vi "周期设置_多参数.vi"() -> ()   [LabVIEW 2016, in "斯坦道多参数.lvlib"]
uses:
  <vilib>/Utility/miscctls.llb/LVPointTypeDef.ctl
  <vilib>/Utility/config.llb/NI_LVConfig.lvlib
panel:
  in  "运行周期":T1
  # "运行模式："
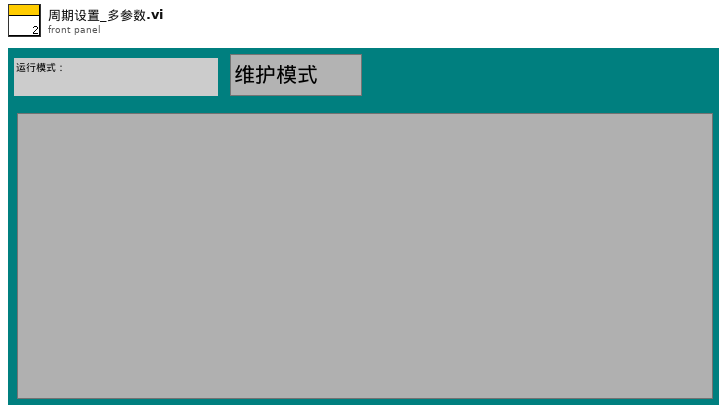
[diagram p1: front panel]
types:
  T1 = cluster{"运行模式":enum16{"维护模式", "常规模式", "应急模式", "质控模式"}, "24H周期设置":bool[]}
  T2 = typedef "斯坦道多参数.lvlib/水样测试启动自定义输入参数.ctl" = cluster{"测量模式":enum16{"待机", "水样测试", "标样核查", "零点核查", "跨度核查", "空白测试", "平行样测试", "加标回收", "空白校准", "标样校准", "初始化（清洗）"}, "数据类型":string, "手动启动标记":bool}
  T3 = typedef "LVPointTypeDef.ctl" = cluster{"Horizontal":i16, "Vertical":i16}
  T4 = typedef "NI_LVConfig.lvlib/Config Data RefNum.ctl" = refnum<k1>
  T5 = typedef "LVDateTimeRec.ctl" = cluster{"秒数的小数部分":dbl, "秒":i32, "分":i32, "时":i32, "日":i32, "月":i32, "年":i32, "天数（周）":i32, "天数（年）":i32, "DST":i32}
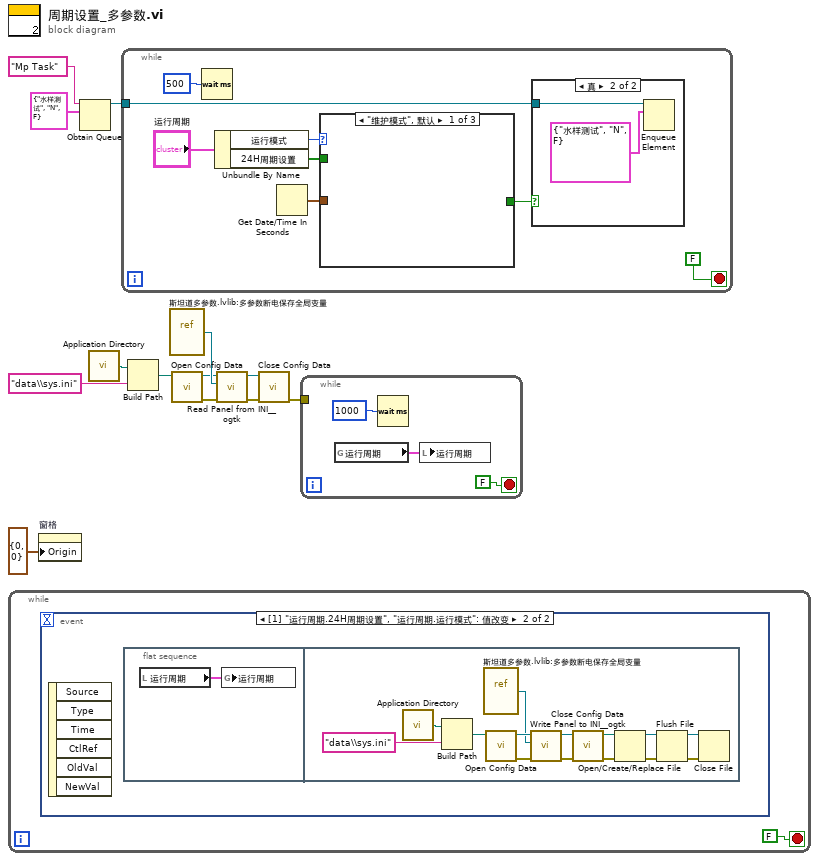
[diagram p0: block diagram]
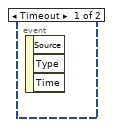
[diagram p2: hidden frame]
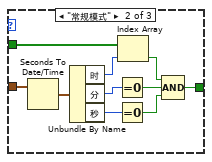
[diagram p4: hidden frame]
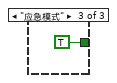
[diagram p5: hidden frame]
diagram:
  n1 = while {
    stop <- FALSE stop-if-true
    n2 = event shown="[1] \"运行周期.24H周期设置\", \"运行周期.运行模式\": 值改变" {
      selector: _ -> [_ _]
      dyn-events: _ -> [_ _]
      timeout: _ -> [_ _]
      event Timeout {
        n3 = event-data() -> ()  [unwired: 1 in, 3 out]
      }
      event "运行周期.24H周期设置", "运行周期.运行模式": Value Change {
        n4 = event-data() -> ()  [unwired: 1 in, 6 out]
        n5 = flat-sequence {
          frame #0 {
            n6 = local read "运行周期"() -> (w15:T1)
            n7 = global write "多参数断电保存全局变量.vi" "运行周期"(w15) -> ()
          }
          frame #1 {
            n8 = call <vilib>:"Application Directory.vi"() -> ("Application Directory"=w29:path)
            n9 = Build Path(base path=w29, name or relative path="data\\sys.ini" ("名称或相对路径")) -> (appended path=w27:path)
            n10 = vi-ref "斯坦道多参数.lvlib:多参数断电保存全局变量.vi"() -> (w25:refnum<vi>)
            n11 = call <vilib>:"Open Config Data.vi"("configuration file path"=w27) -> ("error out"=w23:errorcluster, "refnum"=w26:T4)  [unwired: 8 in, 1 out]
            n12 = call <userlib>:"Write Panel to INI__ogtk.vi"("error in (no error)"=w23, "VI ref"=w25, "refnum"=w26) -> ("error out"=w22:errorcluster, "refnum out"=w24:T4)  [unwired: 7 in]
            n13 = call <vilib>:"Close Config Data.vi"("error in (no error)"=w22, "refnum"=w24) -> ("error out"=w17:errorcluster, "file path"=w16:path)  [unwired: 8 in]
            n14 = Open/Create/Replace File(file path (use dialog)=w16, error in=w17) -> (refnum out=w20:refnum<file>, error out=w21:errorcluster)  [unwired: 4 in, 1 out]
            n15 = Flush File(refnum=w20, error in=w21) -> (refnum out=w19:refnum<file>, error out=w18:errorcluster)
            n16 = Close File(refnum=w19, error in=w18) -> ()  [unwired: 2 out]
          }
        }
      }
    }
  }
  n17 = property on="窗格" class="Pane"("Origin"=T3 {"Horizontal"=0, "Vertical"=0} ("原点")) -> ()  [unwired: 2 in, 2 out]
  n18 = Obtain Queue(name (unnamed)="Mp Task" ("名称（未命名）"), element data type=T2 {"测量模式"=enum."水样测试", "数据类型"="N", "手动启动标记"=FALSE} ("启动参数")) -> (queue out=w1:refnum<queue>)  [unwired: 3 in, 2 out]
  n19 = call <vilib>:"Application Directory.vi"() -> ("Application Directory"=w6:path)
  n20 = while {
    tunnel: w1 -> [w30]
    stop <- FALSE stop-if-true
    n21 = Wait (ms)(milliseconds to wait=u32 500 ("等待时间（毫秒）")) -> ()  [unwired: 1 out]
    n22 = Unbundle By Name("运行周期") -> ("运行模式"=w31:enum16{"维护模式", "常规模式", "应急模式", "质控模式"}, "24H周期设置"=w33:bool[])
    n23 = Get Date/Time In Seconds() -> (seconds since 1Jan1904=w37:timestamp)
    n24 = case shown="\"维护模式\", 默认" w31 {
      tunnel: w37 -> [_ w49 _]
      tunnel: w33 -> [_ w46 _]
      tunnel: [_ w40 TRUE] -> w32
      frame "维护模式", Default {
      }
      frame "常规模式" {
        n25 = Seconds To Date/Time(time stamp (now)=w49) -> (date time rec=w48:T5)  [unwired: 1 in]
        n26 = Unbundle By Name(w48) -> ("时"=w47:i32, "分"=w45:i32, "秒"=w44:i32)
        n27 = Equal To 0?(x=w45) -> (x = 0?=w42:bool)
        n28 = Equal To 0?(x=w44) -> (x = 0?=w41:bool)
        n29 = Index Array(array=w46, index=w47) -> (element=w43:bool)
        n30 = Compound Arithmetic op=AND ("复合运算")(w43, w42, w41) -> (w40:bool)
      }
      frame "应急模式" {
      }
    }
    n31 = case shown="真" w32 {
      tunnel: w30 -> [_ w39]
      frame False {
      }
      frame True {
        n32 = Enqueue Element(queue=w39, element=T2 {"测量模式"=enum."水样测试", "数据类型"="N", "手动启动标记"=FALSE} ("启动参数")) -> ()  [unwired: 2 in, 3 out]
      }
    }
  }
  n33 = Build Path(base path=w6, name or relative path="data\\sys.ini" ("名称或相对路径")) -> (appended path=w8:path)
  n34 = vi-ref "斯坦道多参数.lvlib:多参数断电保存全局变量.vi"() -> (w10:refnum<vi>)
  n35 = call <vilib>:"Open Config Data.vi"("configuration file path"=w8) -> ("error out"=w12:errorcluster, "refnum"=w9:T4)  [unwired: 8 in, 1 out]
  n36 = call <userlib>:"Read Panel from INI__ogtk.vi"("error in (no error)"=w12, "VI ref"=w10, "refnum"=w9) -> ("error out"=w13:errorcluster, "refnum out"=w11:T4)  [unwired: 7 in]
  n37 = call <vilib>:"Close Config Data.vi"("error in (no error)"=w13, "refnum"=w11) -> ("error out"=w5:errorcluster)  [unwired: 8 in, 1 out]
  n38 = while {
    tunnel: w5 -> [_]
    stop <- FALSE stop-if-true
    n39 = global read "多参数断电保存全局变量.vi" "运行周期"() -> (w51:T1)
    n40 = Wait (ms)(milliseconds to wait=u32 1000 ("等待时间（毫秒）")) -> ()  [unwired: 1 out]
    n41 = local write "运行周期"(w51) -> ()
  }
